vi "AOTF_Create_analog_Ports.vi"(0 "Cluster":T1) -> (1 "task out":refnum<k21>, 2 "error out":errorcluster)   [LabVIEW 2009]
uses:
  <vilib>/DAQmx/create/channels.llb/DAQmx Create Channel (AO-Voltage-Basic).vi
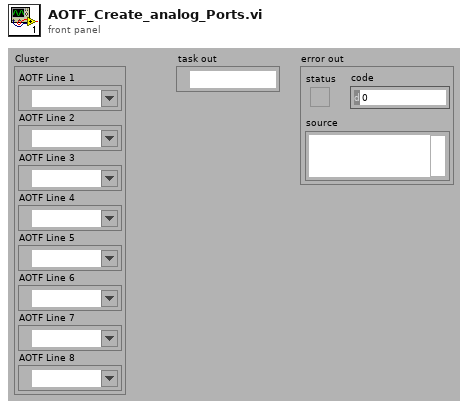
[diagram p1: front panel]
types:
  T1 = cluster{"AOTF Line 1":tag, "AOTF Line 2":tag, "AOTF Line 3":tag, "AOTF Line 4":tag, "AOTF Line 5":tag, "AOTF Line 6":tag, "AOTF Line 7":tag, "AOTF Line 8":tag}
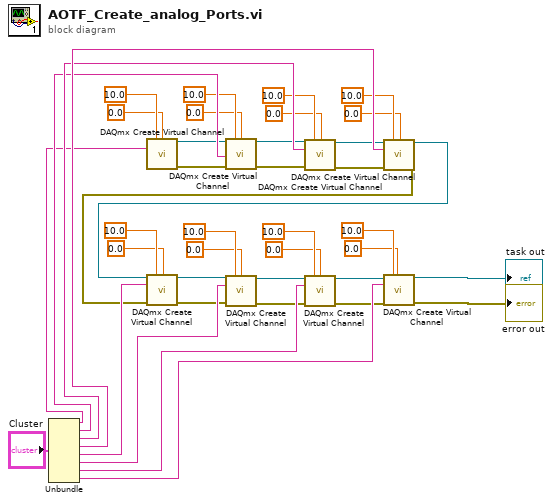
[diagram p0: block diagram]
diagram:
  n1 = Unbundle("Cluster") -> ("AOTF Line 1"=w34:tag, "AOTF Line 2"=w35:tag, "AOTF Line 3"=w36:tag, "AOTF Line 4"=w37:tag, "AOTF Line 5"=w38:tag, "AOTF Line 6"=w39:tag, "AOTF Line 7"=w40:tag, "AOTF Line 8"=w41:tag)
  n2 = call-poly <vilib>:"DAQmx Create Virtual Channel.vi"("maximum value"=10.0, "minimum value"=0.0, "physical channels"=w34) -> ("task out"=w30:refnum<k21>, "error out"=w29:errorcluster)  [unwired: 6 in, 5 out]
  n3 = call-poly <vilib>:"DAQmx Create Virtual Channel.vi"("task in"=w30, "maximum value"=10.0, "minimum value"=0.0, "physical channels"=w35, "error in"=w29) -> ("task out"=w27:refnum<k21>, "error out"=w28:errorcluster)  [unwired: 4 in, 5 out]
  n4 = call-poly <vilib>:"DAQmx Create Virtual Channel.vi"("task in"=w27, "maximum value"=10.0, "minimum value"=0.0, "physical channels"=w36, "error in"=w28) -> ("task out"=w25:refnum<k21>, "error out"=w26:errorcluster)  [unwired: 4 in, 5 out]
  n5 = call-poly <vilib>:"DAQmx Create Virtual Channel.vi"("task in"=w25, "maximum value"=10.0, "minimum value"=0.0, "physical channels"=w37, "error in"=w26) -> ("task out"=w24:refnum<k21>, "error out"=w23:errorcluster)  [unwired: 4 in, 5 out]
  n6 = call-poly <vilib>:"DAQmx Create Virtual Channel.vi"("task in"=w24, "maximum value"=10.0, "minimum value"=0.0, "physical channels"=w38, "error in"=w23) -> ("task out"=w17:refnum<k21>, "error out"=w18:errorcluster)  [unwired: 4 in, 5 out]
  n7 = call-poly <vilib>:"DAQmx Create Virtual Channel.vi"("task in"=w17, "maximum value"=10.0, "minimum value"=0.0, "physical channels"=w39, "error in"=w18) -> ("task out"=w19:refnum<k21>, "error out"=w20:errorcluster)  [unwired: 4 in, 5 out]
  n8 = call-poly <vilib>:"DAQmx Create Virtual Channel.vi"("task in"=w19, "maximum value"=10.0, "minimum value"=0.0, "physical channels"=w40, "error in"=w20) -> ("task out"=w21:refnum<k21>, "error out"=w22:errorcluster)  [unwired: 4 in, 5 out]
  n9 = call-poly <vilib>:"DAQmx Create Virtual Channel.vi"("task in"=w21, "maximum value"=10.0, "minimum value"=0.0, "physical channels"=w41, "error in"=w22) -> ("task out"=→"task out":refnum<k21>, "error out"=→"error out":errorcluster)  [unwired: 4 in, 5 out]
